vi "SUB_REBOOT_Telnet_Formal.vi"() -> (1 "Telnet Ok ?":bool, 2 "msg out":string, 3 "telnet connection out":T1)   [LabVIEW 2011]
uses:
  <vilib>/addons/internet/telnet/telnet.llb/Telnet Session.ctl
panel:
  out "data out":string
  out "Found":bool
  # "Step1:¥ýtelnet log in\nStep2:get root authority\nStep3:REBOOT"
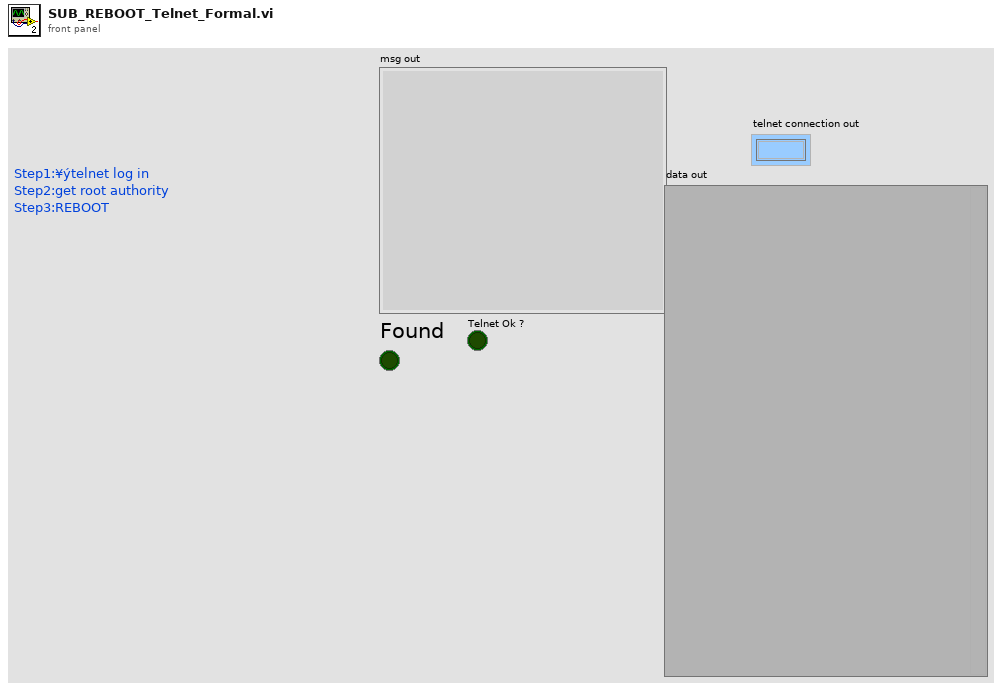
[diagram p1: front panel]
types:
  T1 = typedef "Telnet Session.ctl" = refnum<k1>
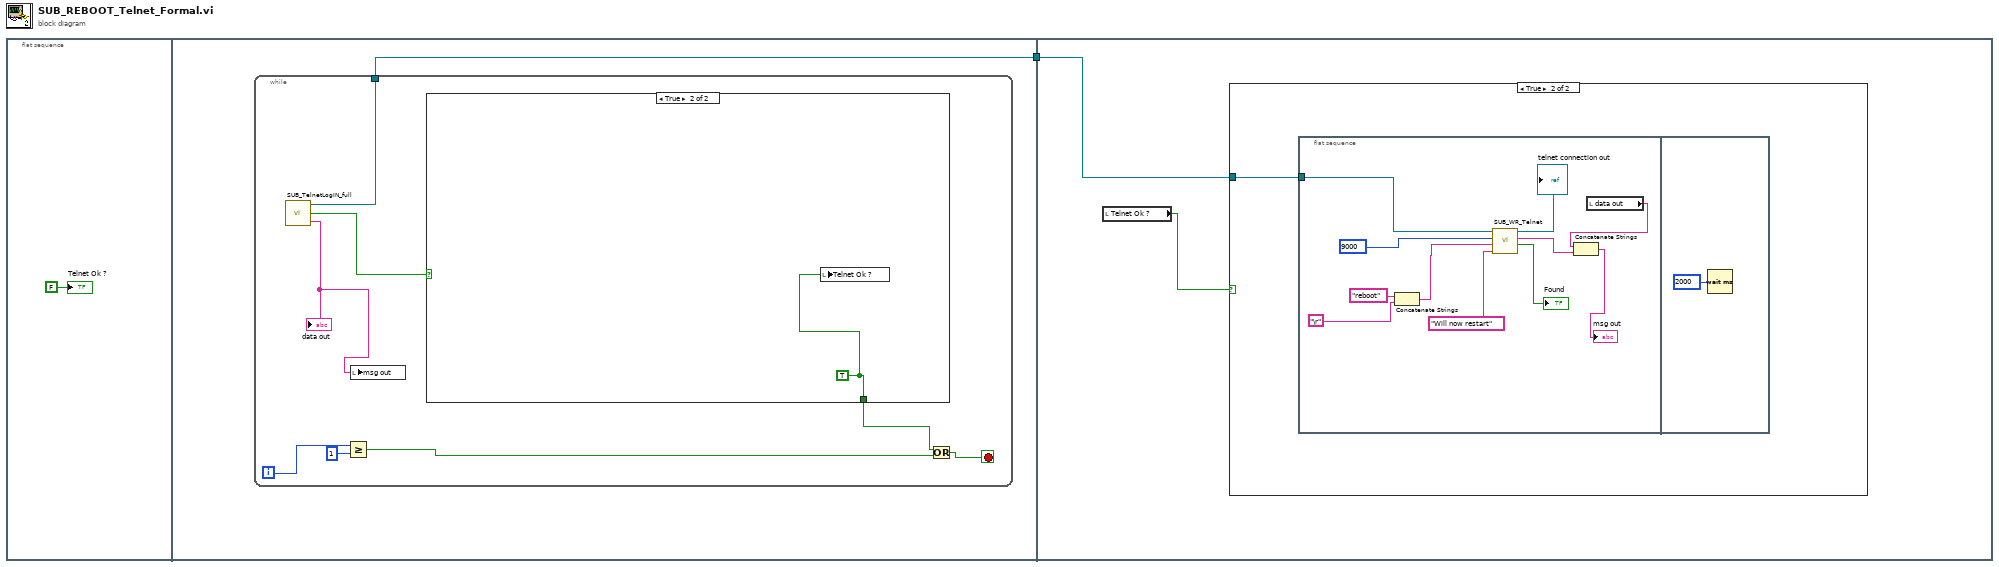
[diagram p0: block diagram]
diagram:
  n1 = flat-sequence {
    tunnel: [w3] -> w1
    tunnel: w1 -> [w13]
    frame #0 {
      "Telnet Ok ?" <- FALSE
    }
    frame #1 {
      n2 = while {
        tunnel: [w11] -> w3
        i -> [w7]
        stop <- w9 stop-if-true
        n3 = call "SUB_TelnetLogIN_full.vi"() -> ("telnet connection"=w11:T1, "Pass ?"=w10:bool, "data out"=w4:string)  [unwired: 2 in]
        "data out" <- w4
        n4 = Greater Or Equal?(x=w7, y=1) -> (x >= y?=w5:bool)
        n5 = local write "msg out"(w4) -> ()
        n6 = case shown="True" w10 {
          tunnel: [_ w12] -> w8
          frame False {
          }
          frame True {
            w12 = TRUE
            n7 = local write "Telnet Ok ?"(w12) -> ()
          }
        }
        n8 = Or(x=w8, y=w5) -> (x .or. y?=w9:bool)
      }
    }
    frame #2 {
      n9 = local read "Telnet Ok ?"() -> (w14:bool)
      n10 = case shown="True" w14 {
        tunnel: w13 -> [_ w15]
        frame False {
        }
        frame True {
          n11 = flat-sequence {
            tunnel: w15 -> [w20]
            frame #0 {
              n12 = Concatenate Strings("reboot" ("string"), "\r") -> (w24:string)
              n13 = call "SUB_WR_Telnet.vi"("Find this String"="Will now restart", "data in"=w24, "timeout ms"=9000, "telnet connection"=w20) -> ("Found"=→"Found":bool, "msg out"=w18:string, "telnet connection out"=→"telnet connection out":T1)  [unwired: 1 in]
              n14 = local read "data out"() -> (w17:string)
              n15 = Concatenate Strings(w17, w18) -> (→"msg out":string)
            }
            frame #1 {
              n16 = Wait (ms)(milliseconds to wait=u32 2000) -> ()  [unwired: 1 out]
            }
          }
        }
      }
    }
  }
